vi "Set Config INI PATH.vi"(3 "error in (no error)":errorcluster, 5 "reference":refnum<vi>) -> (0 "error out":errorcluster, 1 "appended path":path)   [LabVIEW 2025]
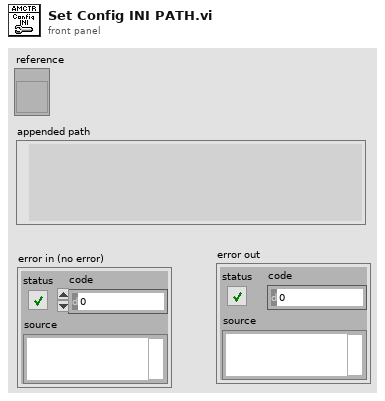
[diagram p1: front panel]
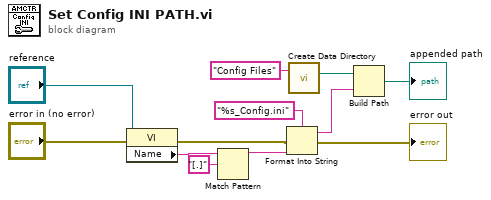
[diagram p0: block diagram]
diagram:
  n1 = property class="VI"(reference="reference", error in="error in (no error)") -> (error out=w10:errorcluster, "Name"=w9:string)  [unwired: 1 out]
  n2 = Match Pattern(string=w9, regular expression="[.]" ("search string")) -> (before substring=w8:string)  [unwired: 1 in, 3 out]
  n3 = Format Into String(format string="%s_Config.ini", error in=w10, w8) -> (resulting string=w6:string, error out=→"error out":errorcluster)  [unwired: 1 in]
  n4 = call "Create Data Directory.vi"("Folder Name"="Config Files") -> ("Path"=w12:path)  [unwired: 2 in]
  n5 = Build Path(base path=w12, name or relative path=w6) -> (appended path=→"appended path":path)
